vi "Cast Data to UI.vi"(4 "Cluster":T1={"Closed Loop Enabled"=TRUE, "Proportional valve 1"=0.0, "Proportional valve 2"=0.0, "Plant Control Variables"={"Tank 1 Level"=0.0, "Tank 2 Level"=0.0, "Tank 3 Level"=0.0, "Tank 4 Level"=0.0, "Pump 1"=0.0, "Pump 2"=0.0}, "Setpoints"={"Setpoint tank 1"=0.0, "Setpoint tank 2"=0.0}}) -> (0 "Pump Voltage":dbl[][](array[numeric]), 1 "Tank Level":dbl[][](array[numeric]), 2 "Graphic Tank Data":T2)   [LabVIEW 2018]
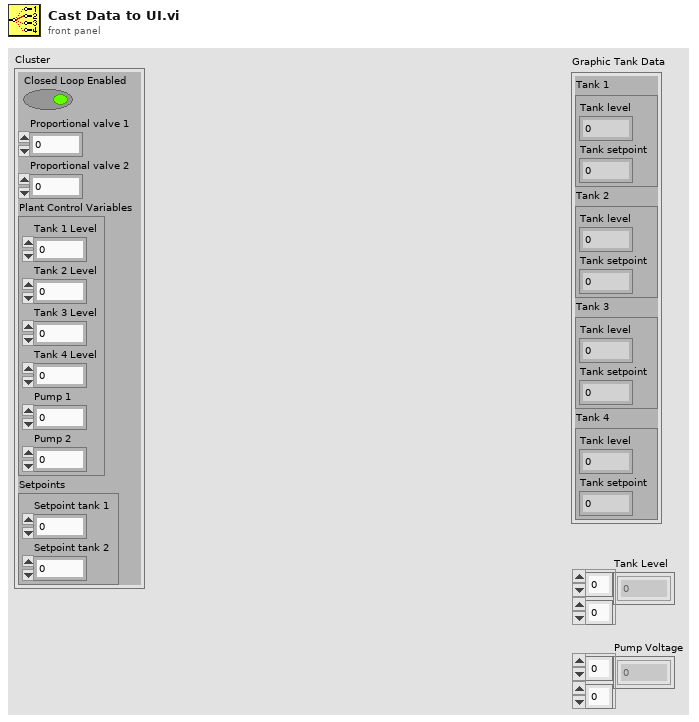
[diagram p1: front panel]
types:
  T1 = cluster{"Closed Loop Enabled":bool, "Proportional valve 1":dbl, "Proportional valve 2":dbl, "Plant Control Variables":cluster{"Tank 1 Level":dbl, "Tank 2 Level":dbl, "Tank 3 Level":dbl, "Tank 4 Level":dbl, "Pump 1":dbl, "Pump 2":dbl}, "Setpoints":cluster{"Setpoint tank 1":dbl, "Setpoint tank 2":dbl}}
  T2 = cluster{"Tank 1":cluster{"Tank level":dbl, "Tank setpoint":dbl}, "Tank 2":cluster{"Tank level":dbl, "Tank setpoint":dbl}, "Tank 3":cluster{"Tank level":dbl, "Tank setpoint":dbl}, "Tank 4":cluster{"Tank level":dbl, "Tank setpoint":dbl}}
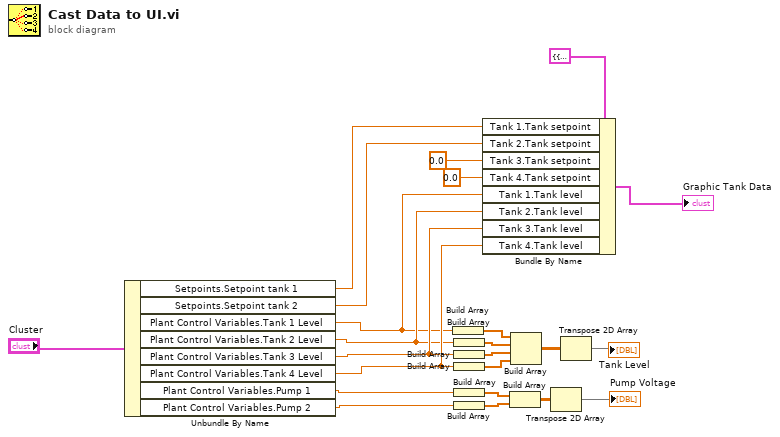
[diagram p0: block diagram]
diagram:
  n1 = Unbundle By Name("Cluster") -> ("Setpoints.Setpoint tank 1"=w6:dbl, "Setpoints.Setpoint tank 2"=w5:dbl, "Plant Control Variables.Tank 1 Level"=w9:dbl, "Plant Control Variables.Tank 2 Level"=w10:dbl, "Plant Control Variables.Tank 3 Level"=w11:dbl, "Plant Control Variables.Tank 4 Level"=w12:dbl, "Plant Control Variables.Pump 1"=w13:dbl, "Plant Control Variables.Pump 2"=w14:dbl)
  n2 = Build Array(w9) -> (w18:dbl[])
  n3 = Build Array(w10) -> (w16:dbl[])
  n4 = Build Array(w11) -> (w17:dbl[])
  n5 = Build Array(w12) -> (w19:dbl[])
  n6 = Build Array(w13) -> (w21:dbl[])
  n7 = Build Array(w14) -> (w22:dbl[])
  n8 = Bundle By Name(cluster=T2 {"Tank 1"={"Tank level"=0.0, "Tank setpoint"=0.0}, "Tank 2"={"Tank level"=0.0, "Tank setpoint"=0.0}, "Tank 3"={"Tank level"=0.0, "Tank setpoint"=0.0}, "Tank 4"={"Tank level"=0.0, "Tank setpoint"=0.0}} ("Graphic Tank Data"), "Tank 1.Tank setpoint"=w6, "Tank 2.Tank setpoint"=w5, "Tank 3.Tank setpoint"=0.0, "Tank 4.Tank setpoint"=0.0, "Tank 1.Tank level"=w9, "Tank 2.Tank level"=w10, "Tank 3.Tank level"=w11, "Tank 4.Tank level"=w12) -> (→"Graphic Tank Data":T2)
  n9 = Build Array(w21, w22) -> (w23:dbl[][])
  n10 = Build Array(w18, w16, w17, w19) -> (w20:dbl[][])
  n11 = Transpose 2D Array(2D array=w23) -> (transposed array=→"Pump Voltage":dbl[][])
  n12 = Transpose 2D Array(2D array=w20) -> (transposed array=→"Tank Level":dbl[][])
